vi "Initalize.vi"(8 "error in (no error)":errorcluster, 9 "Section":string, 10 "Config Path":path, 11 "Motion Controller in":refnum<class "FINE SIM Motion Axis.lvclass">) -> (0 "error out":errorcluster, 3 "Motion Controller out":refnum<class "FINE SIM Motion Axis.lvclass">)   [LabVIEW 2022 SP3, in "FINE SIM Motion Axis.lvclass"]
uses:
  FINE SIM Motion Axis.lvclass
  C:/XY Stage/XY Stage/Framework/Base/Base.lvclass
  TypeDefs/Homing Status.ctl
  TypeDefs/Axis Data.ctl
  TypeDefs/Axis Parameters.ctl
  TypeDefs/Settings.ctl
  TypeDefs/Axis Settings.ctl
  Framework/Base/Base.lvclass/Base.ctl
  FINE SIM Motion Axis.lvclass/FINE SIM Motion Axis.ctl
  Framework/Base/Accessors/Write Config Path.vi
  Framework/Base/Accessors/Write Section.vi
  Accessors/Read Sim Axis Data.vi
  Accessors/Write Sim Axis Data.vi
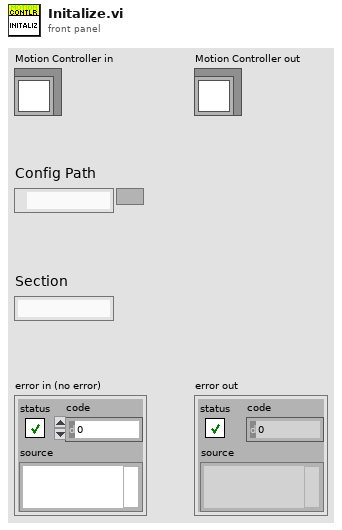
[diagram p1: front panel]
types:
  T1 = typedef "FINE SIM Motion Axis.lvclass/Axis Data.ctl" = cluster{"Axis Parameters":T2, "Time Stamp":timestamp, "Settings":T4}
  T2 = typedef "FINE SIM Motion Axis.lvclass/Axis Parameters.ctl" = cluster{"Moving":bool, "Homed":bool, "Desired Position":dbl, "Current Positon":dbl, "Current Speed":dbl, "Home Status":T3}
  T3 = typedef "FINE SIM Motion Axis.lvclass/Homing Status.ctl" = enum16{"Idle", "Inital Home Motion", "Final Home Motion", "Done Homing"}
  T4 = typedef "FINE SIM Motion Axis.lvclass/Settings.ctl" = cluster{"Axis Name":string, "Axis Settings":T5}
  T5 = typedef "FINE SIM Motion Axis.lvclass/Axis Settings.ctl" = cluster{"Speed":dbl, "Acceleration":dbl}
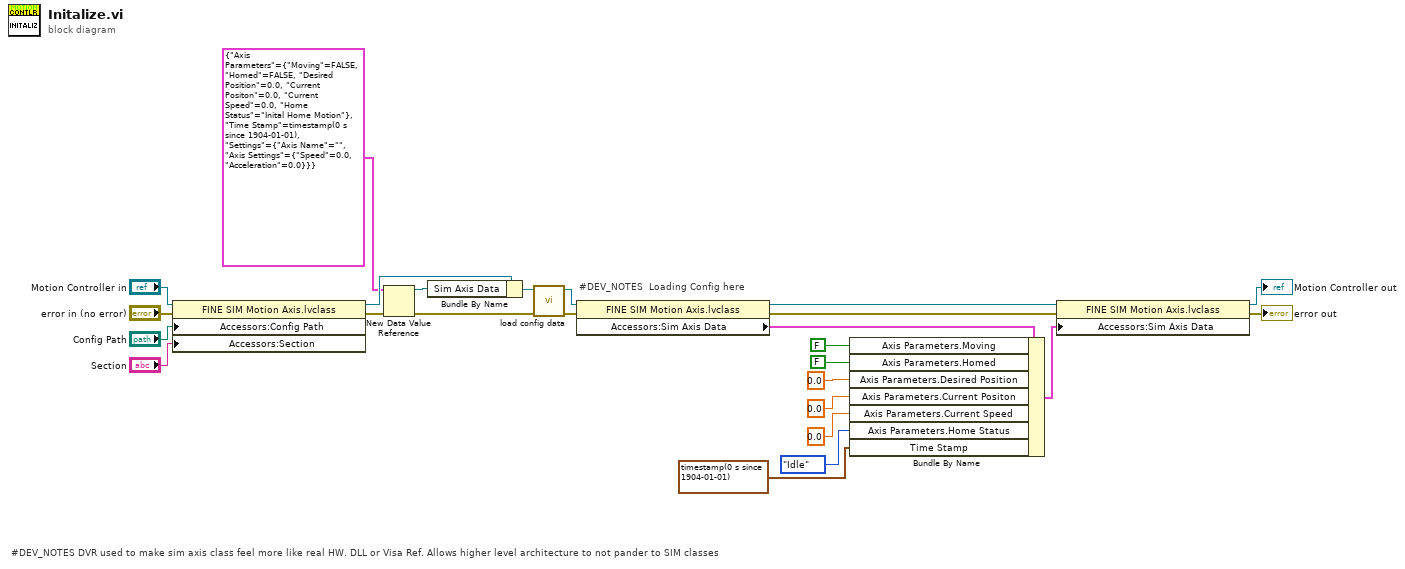
[diagram p0: block diagram]
diagram:
  # "#DEV_NOTES  Loading Config here"
  # "#DEV_NOTES DVR used to make sim axis class feel more like real HW. DLL or Visa Ref. Allows higher level architecture to not pander to SIM classes"
  n1 = property class="FINE SIM Motion Axis.lvclass"(reference="Motion Controller in", error in="error in (no error)", "Accessors:Config Path"="Config Path", "Accessors:Section"="Section") -> (reference out=w23:refnum<class "FINE SIM Motion Axis.lvclass">, error out=w12:errorcluster)
  n2 = New Data Value Reference(data value=T1 {"Axis Parameters"={"Moving"=FALSE, "Homed"=FALSE, "Desired Position"=0.0, "Current Positon"=0.0, "Current Speed"=0.0, "Home Status"=enum."Inital Home Motion"}, "Time Stamp"=timestamp(0 s since 1904-01-01), "Settings"={"Axis Name"="", "Axis Settings"={"Speed"=0.0, "Acceleration"=0.0}}} ("output cluster"), error in=w12) -> (data value reference=w13:refnum<data-value>, error out=w2:errorcluster)
  n3 = Bundle By Name(cluster=w23, "Sim Axis Data"=w13) -> (w4:refnum<class "FINE SIM Motion Axis.lvclass">)
  n4 = call-dynamic "load config data.vi"("error in (no error)"=w2, "FINE SIM Motion Axis in"=w4) -> ("error out"=w1:errorcluster, "FINE SIM Motion Axis out"=w3:refnum<class "FINE SIM Motion Axis.lvclass">)  [unwired: 8 in]
  n5 = property class="FINE SIM Motion Axis.lvclass"(reference=w3, error in=w1) -> (reference out=w9:refnum<class "FINE SIM Motion Axis.lvclass">, error out=w11:errorcluster, "Accessors:Sim Axis Data"=w7:T1)
  n6 = Bundle By Name(cluster=w7, "Axis Parameters.Moving"=FALSE, "Axis Parameters.Homed"=FALSE, "Axis Parameters.Desired Position"=0.0, "Axis Parameters.Current Positon"=0.0, "Axis Parameters.Current Speed"=0.0, "Axis Parameters.Home Status"=Homing_Status."Idle", "Time Stamp"=timestamp(0 s since 1904-01-01)) -> (w6:T1)
  n7 = property class="FINE SIM Motion Axis.lvclass"(reference=w9, error in=w11, "Accessors:Sim Axis Data"=w6) -> (reference out=→"Motion Controller out":refnum<class "FINE SIM Motion Axis.lvclass">, error out=→"error out":errorcluster)
